vi "Show Panel.vi"(8 "error in (no error)":errorcluster) -> (0 "error out":errorcluster)   [LabVIEW 2019, in "ContextHelp.lvlib"]
doc: "Send the Show Panel request to the Module's Main.vi.\n_____\nBased on DQMH Project Template 6.1.0.94.\n____\nPantherLAB Templates 1.0.0.5\nCopyright (c) 2022, PantherLAB"
uses:
  ContextHelp.lvlib
  Show Panel Argument--cluster.ctl
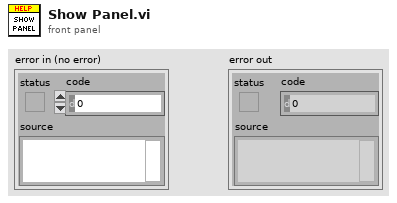
[diagram p1: front panel]
types:
  T1 = typedef "ContextHelp.lvlib/Show Panel Argument--cluster.ctl" = cluster{"Show Panel?":bool}
  T2 = typedef "ContextHelp.lvlib/Request Events--cluster.ctl" = cluster{"Stop Module":refnum<user-event>, "Show Panel":refnum<user-event>, "Hide Panel":refnum<user-event>, "Get Module Execution Status":refnum<user-event>, "Show Diagram":refnum<user-event>, "Wake up Helper Loop":refnum<user-event>, "Put Helper Loop to Sleep":refnum<user-event>, "Draw Panel Into Subpanel":refnum<user-event>, "Remove Panel from Subpanel":refnum<user-event>, "Refresh Panther Dashboard Broadcasts":refnum<user-event>}
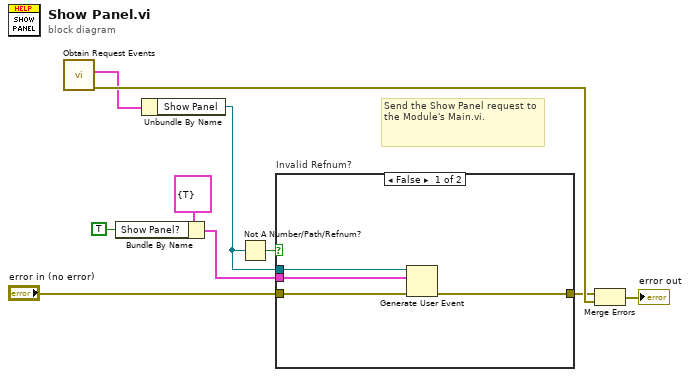
[diagram p0: block diagram]
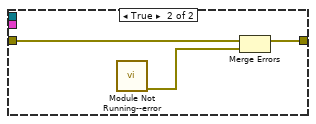
[diagram p2: hidden frame]
diagram:
  # "Send the Show Panel request to the Module's Main.vi."
  n1 = call "Obtain Request Events.vi"() -> ("error out"=w9:errorcluster, "ContextHelp Request Events"=w8:T2)  [unwired: 10 in]
  n2 = Bundle By Name(cluster=T1 {"Show Panel?"=TRUE} ("Show Panel Argument"), "Show Panel?"=TRUE) -> (w2:T1)
  n3 = Unbundle By Name(w8) -> ("Show Panel"=w6:refnum<user-event>)
  n4 = Not A Number/Path/Refnum?(number/path/refnum=w6) -> (NaN/Path/Refnum?=w7:bool)
  n5 = case "Invalid Refnum?" shown="False" w7 {
    tunnel: "error in (no error)" -> [w14 w17]
    tunnel: [w13 w16] -> w4
    tunnel: w6 -> [w12 _]
    tunnel: w2 -> [w11 _]
    frame False {
      n6 = Generate User Event(user event=w12, event data cluster=w11, error in=w14) -> (error out=w13:errorcluster)  [unwired: 1 in, 1 out]
    }
    frame True {
      n7 = call "Module Not Running--error.vi"() -> ("error out"=w15:errorcluster)  [unwired: 11 in]
      n8 = Merge Errors(w17, w15) -> (w16:errorcluster)
    }
  }
  n9 = Merge Errors(w4, w9) -> (→"error out":errorcluster)
